vi "PictureType.vi"(1 "Camera Angle":dbl, 2 "Grating#":i32) -> (0 "GS_picture_tab":u16)   [LabVIEW 2015]
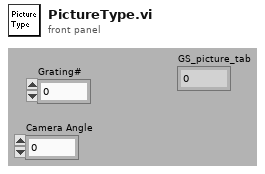
[diagram p1: front panel]
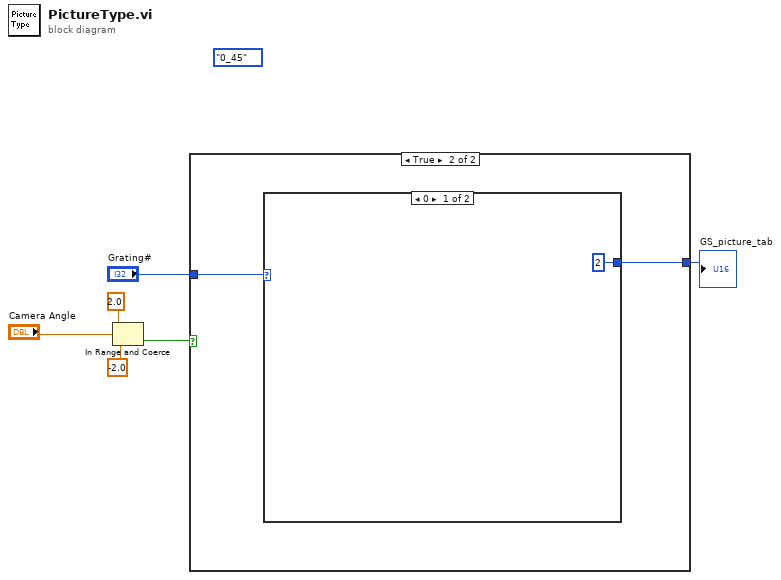
[diagram p0: block diagram]
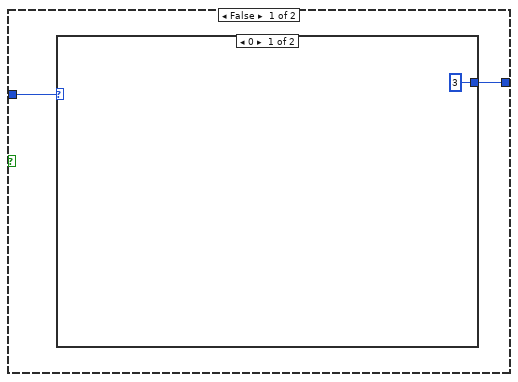
[diagram p2: hidden frame]
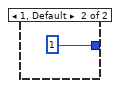
[diagram p3: hidden frame]
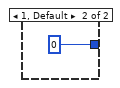
[diagram p4: hidden frame]
diagram:
  (unwired) enum32{"1_45", "1_0", "0_0", "0_45"}."0_45" ("GS_picture_tab")
  n1 = In Range and Coerce(upper limit=2.0, x="Camera Angle", lower limit=-2.0 ("x")) -> (In Range?=w3:bool)  [unwired: 1 out]
  n2 = case shown="True" w3 {
    tunnel: "Grating#" -> [w8 w12]
    tunnel: [w7 w11] -> w1
    frame False {
      n3 = case shown="0" w8 {
        tunnel: [u16 3 ("GS_picture_tab") u16 1 ("GS_picture_tab")] -> w7
        frame 0 {
        }
        frame 1, Default {
        }
      }
    }
    frame True {
      n4 = case shown="0" w12 {
        tunnel: [u16 2 ("GS_picture_tab") u16 0 ("GS_picture_tab")] -> w11
        frame 0 {
        }
        frame 1, Default {
        }
      }
    }
  }
  "GS_picture_tab" <- w1
